vi "Write Active Path.vi"(8 "error in (no error)":errorcluster, 10 "Path Settings.lvclass":refnum<class "Path Settings.lvclass">, 11 "Setting Database in":refnum<class "Setting Database.lvclass">) -> (0 "error out":errorcluster, 3 "Setting Database out":refnum<class "Setting Database.lvclass">)   [LabVIEW 2019, in "Setting Database.lvclass"]
uses:
  Setting Database.lvclass
  Path Settings/Path Settings.lvclass
  C:/Users/Albro/Documents/GitHub/AFM-Lithography/lvsrc/Classes/Settings/ObjectSettings/ObjectSettings.lvclass
  Setting Database.lvclass/Setting Database.ctl
  ObjectSettings/ObjectSettings.lvclass/ObjectSettings.ctl
  ObjectSettings/Accessors/Read Enabled.vi
  ObjectSettings/Accessors/Write Enabled.vi
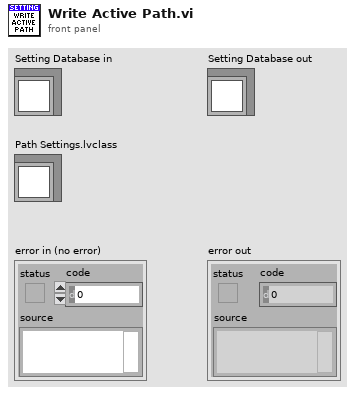
[diagram p1: front panel]
types:
  T1 = cluster{"Path":i32, "Funnel":i32, "Rectangle":i32, "Dot":i32}
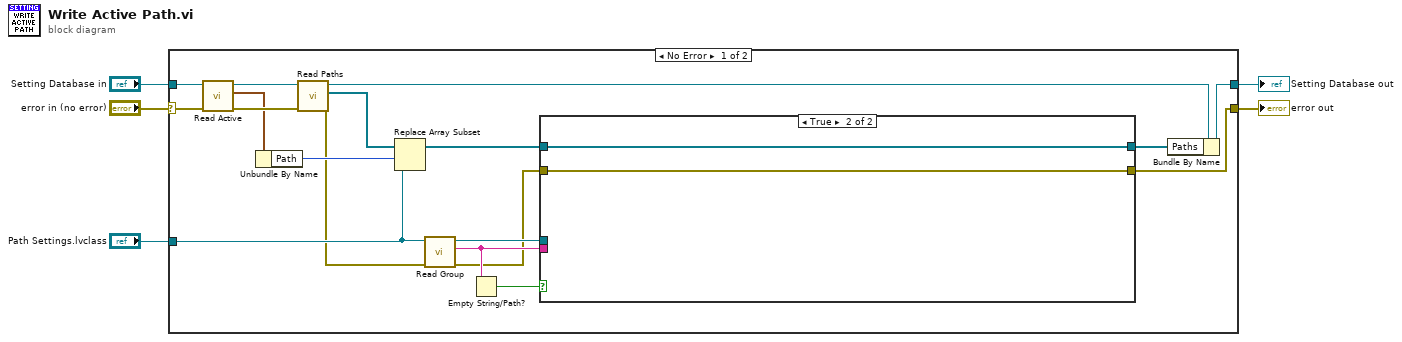
[diagram p0: block diagram]
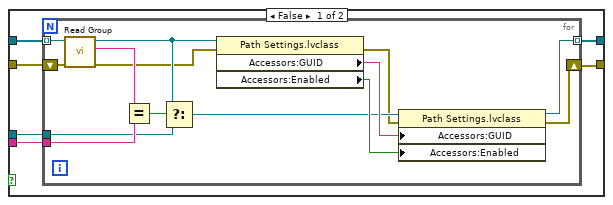
[diagram p2: hidden frame]
diagram:
  n1 = case shown="No Error" "error in (no error)" {
    selector: "error in (no error)" -> [w22 w47]
    tunnel: [w6 w47] -> w4
    tunnel: [w21 w46] -> w2
    tunnel: "Setting Database in" -> [w17 w46]
    tunnel: "Path Settings.lvclass" -> [w14 _]
    frame No Error {
      n2 = call "Read Active.vi"("error in (no error)"=w22, "Setting Database in"=w17) -> ("error out"=w23:errorcluster, "Active"=w16:T1, "Setting Database out"=w18:refnum<class "Setting Database.lvclass">)  [unwired: 7 in]
      n3 = Unbundle By Name(w16) -> ("Path"=w15:i32)
      n4 = call "Read Paths.vi"("error in (no error)"=w23, "Setting Database in"=w18) -> ("error out"=w7:errorcluster, "Paths"=w19:refnum<class "Path Settings.lvclass">[], "Setting Database out"=w20:refnum<class "Setting Database.lvclass">)  [unwired: 7 in]
      n5 = Replace Array Subset(array=w19, new element=w14, index=w15) -> (w13:refnum<class "Path Settings.lvclass">[])
      n6 = call-dynamic "Read Group.vi"("error in (no error)"=w7, "ObjectSettings in"=w14) -> ("error out"=w8:errorcluster, "Group"=w10:string, "ObjectSettings out"=w9:refnum<class "Path Settings.lvclass">)  [unwired: 7 in]
      n7 = Empty String/Path?(string/path=w10) -> (empty?=w12:bool)
      n8 = case shown="True" w12 {
        tunnel: w13 -> [w28 w45]
        tunnel: [w26 w45] -> w11
        tunnel: w10 -> [w29 _]
        tunnel: w9 -> [w27 _]
        tunnel: w8 -> [w25 w44]
        tunnel: [w24 w44] -> w6
        frame False {
          n9 = for {
            tunnel: w29 -> [w41]
            tunnel: w28 -> [w43] mode=indexing
            tunnel: w27 -> [w40]
            tunnel: [w38] -> w26 mode=indexing
            shift-right: [w30] -> w24
            shift-left: w25 -> [w31]
            n10 = call-dynamic "Read Group.vi"("error in (no error)"=w31, "ObjectSettings in"=w43) -> ("error out"=w32:errorcluster, "Group"=w42:string, "ObjectSettings out"=w39:refnum<class "Path Settings.lvclass">)  [unwired: 7 in]
            n11 = Equal?(x=w42, y=w41) -> (x = y?=w34:bool)
            n12 = Select(t=w39, s=w34, f=w40) -> (s? t:f=w35:refnum<class "Path Settings.lvclass">)
            n13 = property class="Path Settings.lvclass"(reference=w39, error in=w32) -> (error out=w33:errorcluster, "Accessors:GUID"=w37:string, "Accessors:Enabled"=w36:bool)  [unwired: 1 out]
            n14 = property class="Path Settings.lvclass"(reference=w35, error in=w33, "Accessors:GUID"=w37, "Accessors:Enabled"=w36) -> (reference out=w38:refnum<class "Path Settings.lvclass">, error out=w30:errorcluster)
          }
        }
        frame True {
        }
      }
      n15 = Bundle By Name(cluster=w20, "Paths"=w11) -> (w21:refnum<class "Setting Database.lvclass">)
    }
    frame Error {
    }
  }
  "error out" <- w4
  "Setting Database out" <- w2
